vi "Table-Remove decimal points.vi"(8 "error in (no error)":errorcluster, 10 "NewVal":string[][](array[string]), 11 "OldVal":string[][](array[string])) -> (0 "error out":errorcluster, 2 "NewVal out":string[][](array[string]))   [LabVIEW 2013]
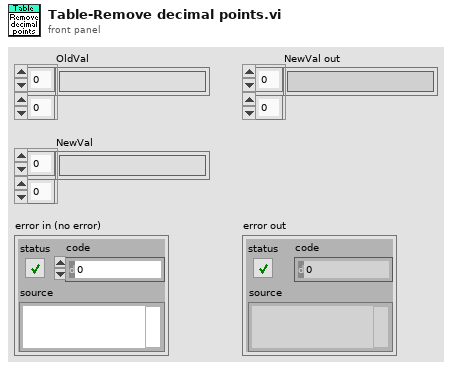
[diagram p1: front panel]
types:
  T1 = typedef "LVRowAndColumnTypeDef.ctl" = cluster{"Row":i32, "Column":i32}
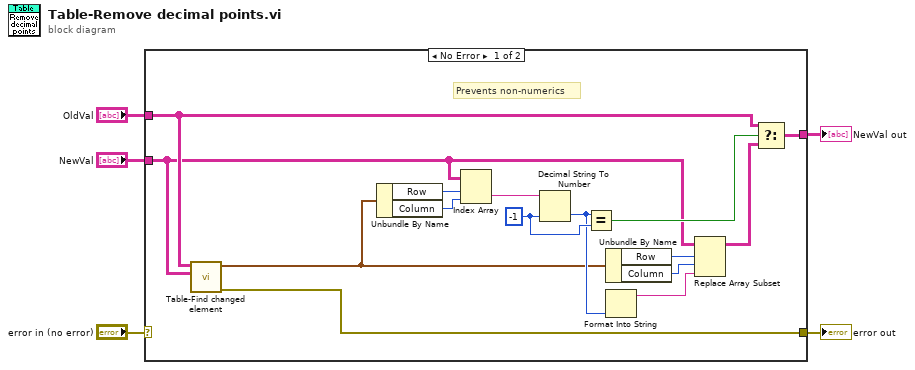
[diagram p0: block diagram]
diagram:
  n1 = case shown="No Error" "error in (no error)" {
    selector: "error in (no error)" -> [_ w21]
    tunnel: [w18 _] -> w5
    tunnel: "OldVal" -> [w11 _]
    tunnel: "NewVal" -> [w8 _]
    tunnel: [w6 w21] -> w1
    frame No Error {
      w20 = -1 ("default (0 I32)")
      # "Prevents non-numerics"
      n2 = call "Table-Find changed element.vi"("Table 2"=w8, "Table 1"=w11) -> ("error out"=w6:errorcluster, "Index of change"=w9:T1)  [unwired: 8 in]
      n3 = Unbundle By Name(w9) -> ("Row"=w15:i32, "Column"=w16:i32)
      n4 = Index Array(array=w8, index (row)=w15, index (col)=w16) -> (element=w17:string)
      n5 = Decimal String To Number(string=w17, default (0L)=w20) -> (number=w10:i32)  [unwired: 1 in, 1 out]
      n6 = Equal?(x=w10, y=w20) -> (x = y?=w19:bool)
      n7 = Unbundle By Name(w9) -> ("Row"=w14:i32, "Column"=w13:i32)
      n8 = Format Into String(w10) -> (resulting string=w12:string)  [unwired: 3 in, 1 out]
      n9 = Replace Array Subset(array=w8, new element=w12, index (row)=w14, index (col)=w13) -> (w7:string[][])
      n10 = Select(t=w11, s=w19, f=w7) -> (s? t:f=w18:string[][])
    }
    frame Error {
    }
  }
  "NewVal out" <- w5
  "error out" <- w1
